vi "AlazarDSPGetNextBufferU16.vi"(4 "error in (no error)":errorcluster, 5 "timeout_ms":u32, 6 "Buffer":u16[](array[numeric]), 7 "Handle":u64) -> (0 "error out":errorcluster, 1 "Return Code":u32, 2 "Buffer":u16[](array[numeric]), 3 "Handle":u64)   [LabVIEW 2018]
doc: "This function returns when the board has received sufficient trigger events to fill the buffer, or the timeout interval has elapsed. To use this function, AlazarBeforeAsyncRead must be called with the ADMA_ALLOC_BUFFERS flag."
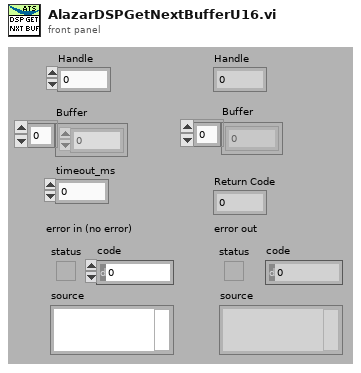
[diagram p1: front panel]
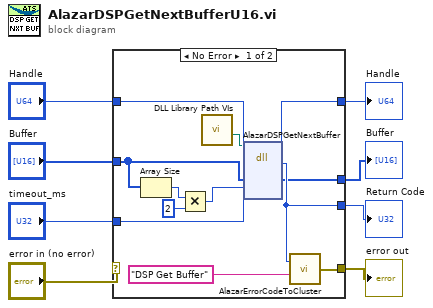
[diagram p0: block diagram]
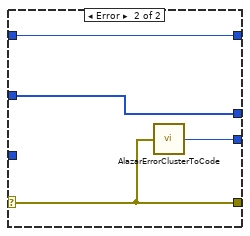
[diagram p2: hidden frame]
diagram:
  n1 = case shown="No Error" "error in (no error)" {
    selector: "error in (no error)" -> [_ w24]
    tunnel: [w17 w24] -> w7
    tunnel: [w19 w23] -> w6
    tunnel: "Handle" -> [w20 w22]
    tunnel: [w16 w22] -> w4
    tunnel: "Buffer" -> [w13 w21]
    tunnel: "timeout_ms" -> [w14 _]
    tunnel: [w15 w21] -> w1
    frame No Error {
      n2 = Array Size(array=w13) -> (size(s)=w12:i32)
      n3 = Multiply(x=w12, y=2) -> (x*y=w10:i32)
      n4 = call "DLL Library Path VIs.vi"() -> ("Alazar"=w9:path)  [unwired: 9 in, 2 out]
      n5 = dll-call lib="C:/Project/SerialSectOCT - FFT GPU/SerialSectOCT/Labview Software/DLL/ATSApi.dll" fn="AlazarDSPGetNextBuffer"(path in=w9, "handle"=w20, "buffer"=w13, "bytesToCopy"=w10, "timeout_ms"=w14) -> ("return type"=w19:u32, "handle"=w16:u64, "buffer"=w15:u16[])  [unwired: 4 in, 2 out]
      n6 = call "AlazarErrorCodeToCluster.vi"("Message"="DSP Get Buffer", "Error Code"=w19) -> ("error out"=w17:errorcluster)
    }
    frame Error {
      n7 = call "AlazarErrorClusterToCode.vi"("error in (no error)"=w24) -> ("Error Code"=w23:u32)
    }
  }
  "Handle" <- w4
  "error out" <- w7
  "Return Code" <- w6
  "Buffer" <- w1
